vi "mupLib Eval example.vi"() -> ()   [LabVIEW 2015]
uses:
  mupLib/mupLibPath.vi
  mupLib/mupCheckError.vi
  <vilib>/Utility/error.llb/Error Cluster From Error Code.vi
  mupLib/mupLib.lvlib
panel:
  out "error out":errorcluster
  out "Array":dbl[](array[numeric])
  in  "c":dbl
  in  "szExpr":string="a*x^2+b*x+c"
  in  "x":dbl
  in  "b":dbl
  in  "a":dbl
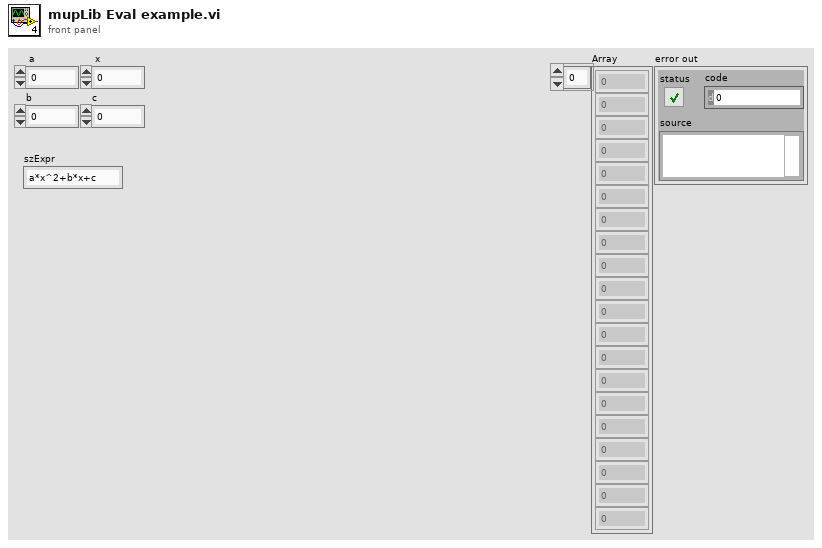
[diagram p1: front panel]
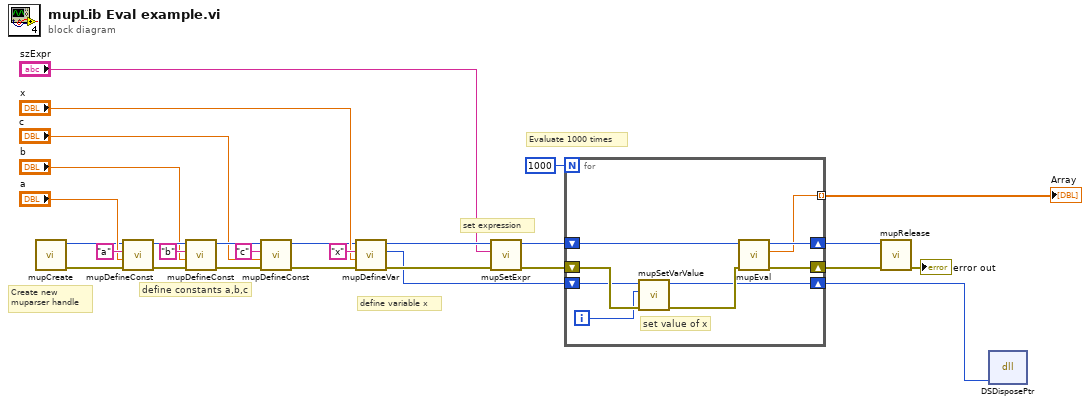
[diagram p0: block diagram]
diagram:
  # "Evaluate 1000 times"
  # "set expression"
  # "define variable x"
  # "define constants a,b,c"
  # "Create new\nmuparser handle"
  n1 = call "mupCreate.vi"() -> ("error out"=w28:errorcluster, "hParser out"=w1:u64)  [unwired: 10 in]
  n2 = call "mupDefineConst.vi"("error in (no error)"=w28, "Value"="a", "constName"="a", "hParser in"=w1) -> ("error out"=w23:errorcluster, "hParser out"=w24:u64)  [unwired: 6 in]
  n3 = call "mupDefineConst.vi"("error in (no error)"=w23, "Value"="b", "constName"="b", "hParser in"=w24) -> ("error out"=w14:errorcluster, "hParser out"=w15:u64)  [unwired: 6 in]
  n4 = call "mupDefineConst.vi"("error in (no error)"=w14, "Value"="c", "constName"="c", "hParser in"=w15) -> ("error out"=w12:errorcluster, "hParser out"=w11:u64)  [unwired: 6 in]
  n5 = call "mupDefineVar.vi"("error in (no error)"=w12, "initValue"="x", "varName"="x", "hParser in"=w11) -> ("error out"=w17:errorcluster, "varAddr"=w7:u64, "hParser out"=w19:u64)  [unwired: 5 in]
  n6 = call "mupSetExpr.vi"("error in (no error)"=w17, "szExpr"="szExpr", "muPar in"=w19) -> ("error out"=w9:errorcluster, "muPar out"=w10:u64)  [unwired: 7 in]
  n7 = for {
    N: 1000 -> [_]
    shift-right: [w31] -> w4
    shift-left: w10 -> [w34]
    shift-right: [w32] -> w3
    shift-left: w9 -> [w37]
    tunnel: [w30] -> w8 mode=indexing
    shift-right: [w29] -> w6
    shift-left: w7 -> [w36]
    i -> [w35]
    # "set value of x"
    n8 = call "mupSetVarValue.vi"("error in (no error)"=w37, "varValue"=w35, "varPtr in"=w36) -> ("error out"=w33:errorcluster, "varPtr out"=w29:u64)  [unwired: 7 in]
    n9 = call "mupEval.vi"("error in (no error)"=w33, "hParser in"=w34) -> ("error out"=w32:errorcluster, "result"=w30:dbl, "hParser out"=w31:u64)  [unwired: 7 in]
  }
  "Array" <- w8
  n10 = call "mupRelease.vi"("error in (no error)"=w3, "hParser in"=w4) -> ("error out"=→"error out":errorcluster)  [unwired: 9 in]
  n11 = dll-call lib="LabVIEW" fn="DSDisposePtr"("ptr"=w6) -> ()  [unwired: 5 in, 2 out]
